vi "Ready to send.vi"(8 "error in (no error)":errorcluster, 11 "Entradas":string[](array[string])) -> (0 "error IO":errorcluster, 1 "Code":string, 2 "Resultante":string[](array[string]), 3 "Is Null?":bool)   [LabVIEW 2018]
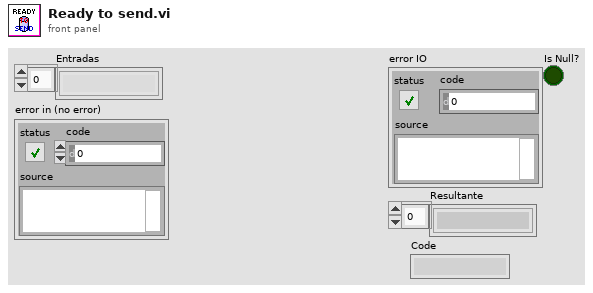
[diagram p1: front panel]
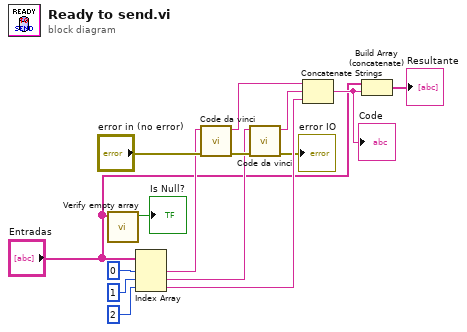
[diagram p0: block diagram]
diagram:
  n1 = call "Verify empty array.vi"("Entradas"="Entradas") -> ("Is Null?"=→"Is Null?":bool)  [unwired: 10 in]
  n2 = Index Array(array="Entradas", index #1=0 ("index"), index #2=1 ("index"), index #3=2 ("index")) -> (element #1=w11:string, element #2=w9:string, element #3=w6:string)
  n3 = call "Code da vinci.vi"("error in (no error)"="error in (no error)", "Cadena entrada"=w11) -> ("error IO"=w10:errorcluster, "Codigo"=w8:string)  [unwired: 8 in]
  n4 = call "Code da vinci.vi"("error in (no error)"=w10, "Cadena entrada"=w9) -> ("error IO"=→"error IO":errorcluster, "Codigo"=w7:string)  [unwired: 8 in]
  n5 = Concatenate Strings(w8, w7, w6) -> (w5:string)
  "Code" <- w5
  n6 = Build Array (concatenate)("Entradas", w5) -> (→"Resultante":string[])
